vi "git_push.vi"(8 "Error In":errorcluster, 10 "Working Directory In":path=path "", 11 "push_button":bool) -> (0 "Error Out":errorcluster, 1 "git push output":string, 2 "Working Directory Out":path, 3 "push_indicator":bool)   [LabVIEW 2026]
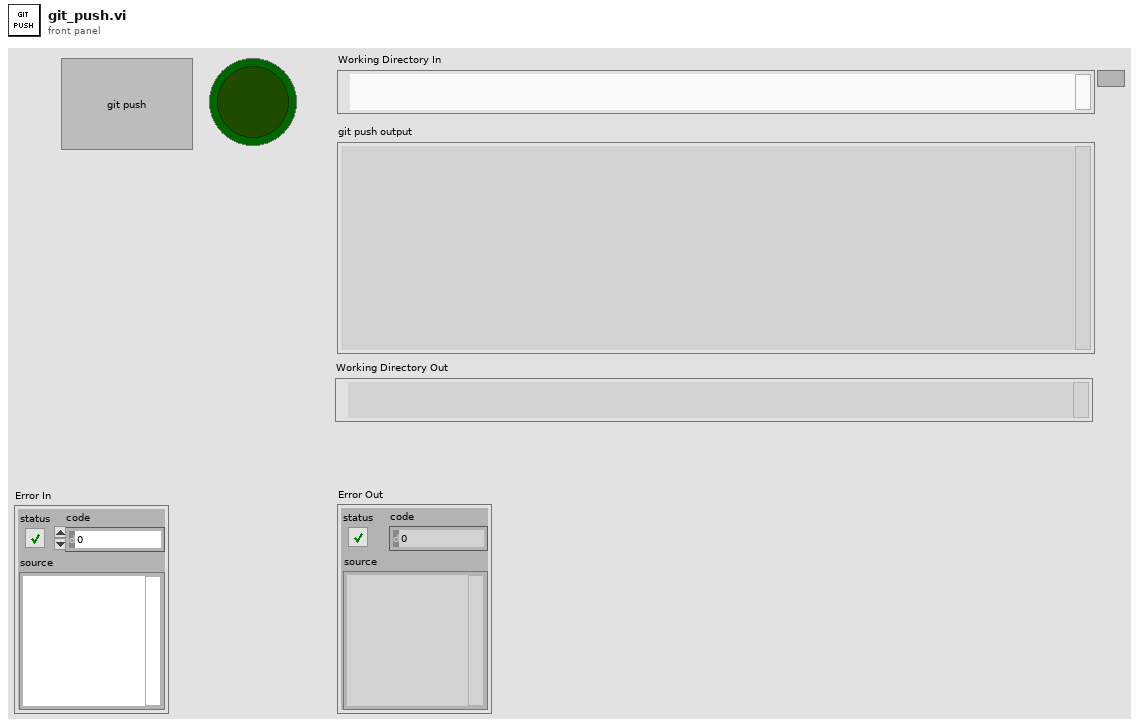
[diagram p1: front panel]
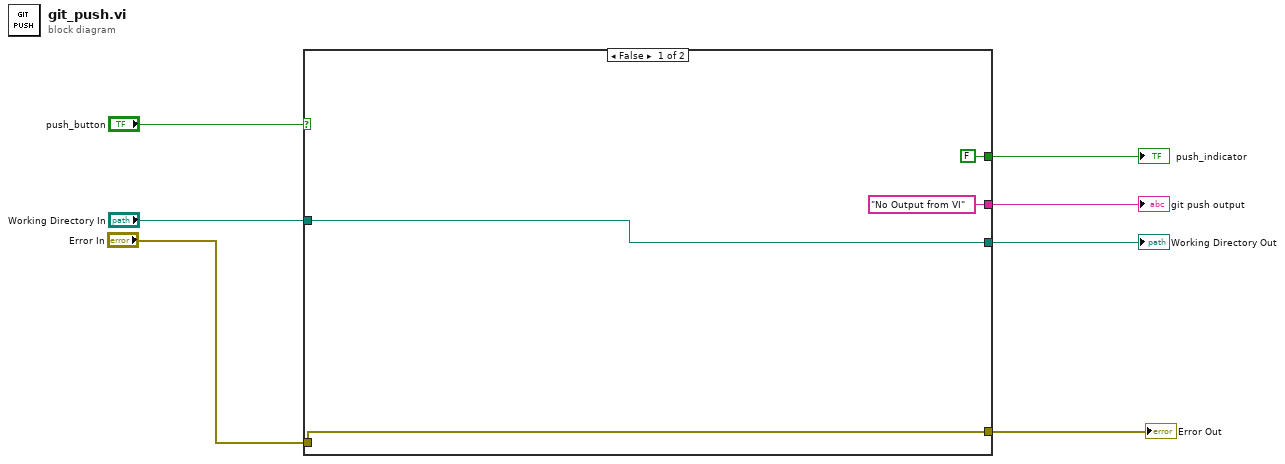
[diagram p0: block diagram]
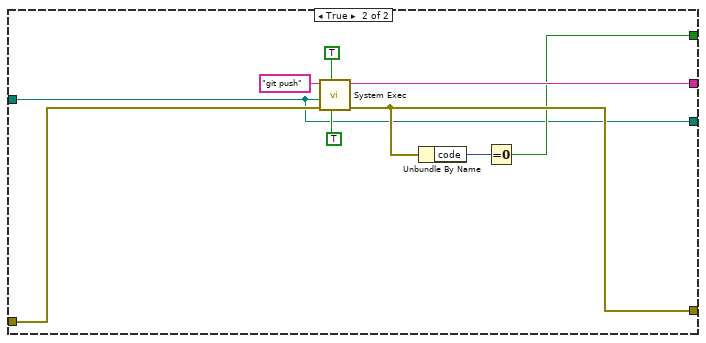
[diagram p2: hidden frame]
diagram:
  n1 = case shown="False" "push_button" {
    tunnel: "Working Directory In" -> [w8 w12]
    tunnel: "Error In" -> [w9 w19]
    tunnel: [w9 w15] -> w5
    tunnel: ["No Output from VI" ("standard output") w17] -> w4
    tunnel: [FALSE w13] -> w3
    tunnel: [w8 w12] -> w1
    frame False {
    }
    frame True {
      n2 = call <vilib>:"System Exec.vi"("run minimized? (F)"=TRUE, "wait until completion? (T)"=TRUE, "error in (no error)"=w19, "working directory"=w12, "command line"="git push") -> ("error out"=w15:errorcluster, "standard output"=w17:string)  [unwired: 3 in, 2 out]
      n3 = Unbundle By Name(w15) -> ("code"=w14:i32)
      n4 = Equal To 0?(x=w14) -> (x = 0?=w13:bool)
    }
  }
  "Error Out" <- w5
  "git push output" <- w4
  "push_indicator" <- w3
  "Working Directory Out" <- w1
